vi "Process_Array.vi"(4 "Image array":dbl[][](array[numeric]), 6 "Base_name":string, 7 "Image In":T4, 8 "Bleed (mm)":dbl, 9 "Step (mm) 2":dbl, 10 "X dim + bleed (mm)":dbl, 11 "Y dim + bleed (mm)":dbl) -> (3 "Image array":dbl[][](array[numeric]), 5 "Image Out":T4)   [LabVIEW 2018]
uses:
  <vilib>/vision/Image Controls.llb/IMAQ Image.ctl
  <vilib>/vision/Pattern Matching.llb/IMAQ Curve Parameters.ctl
  <vilib>/vision/Shape Detection.llb/ShapeDetectionMatchOptions.ctl
  <vilib>/vision/Pattern Matching.llb/IMAQ Match Range Setting.ctl
  <vilib>/Utility/file.llb/Write Delimited Spreadsheet (DBL).vi
  <vilib>/vision/NI_Vision_Development_Module.lvlib
panel:
  in  "Match Options":T1 {"Range Settings"."Match Constraints" items=["Rotation Angle (degrees)", "Scale Factor (%)", "Occlusion (%)"]}
  in  "Curve Parameters":T3={"Extraction Mode"=0, "Edge Threshold"=75, "Edge Filter Size"=1, "Min Length"=25, "Row Search Step Size"=15, "Col Search Step Size"=15, "Max Endpoint Gap"=10, "Closed"=FALSE, "Subpixel"=FALSE} {"Max Endpoint Gap" min=0; "Col Search Step Size" min=1 max=255 step=1; "Row Search Step Size" min=1 max=255 step=1; "Min Length" min=0; "Edge Filter Size" items=["Fine", "Normal", "Controur Tracing"]; "Edge Threshold" min=1 max=65535 step=1; "Extraction Mode" items=["Normal", "Uniform Regions"]}
  out "Number of Matches Returned":i32
  # "Range"
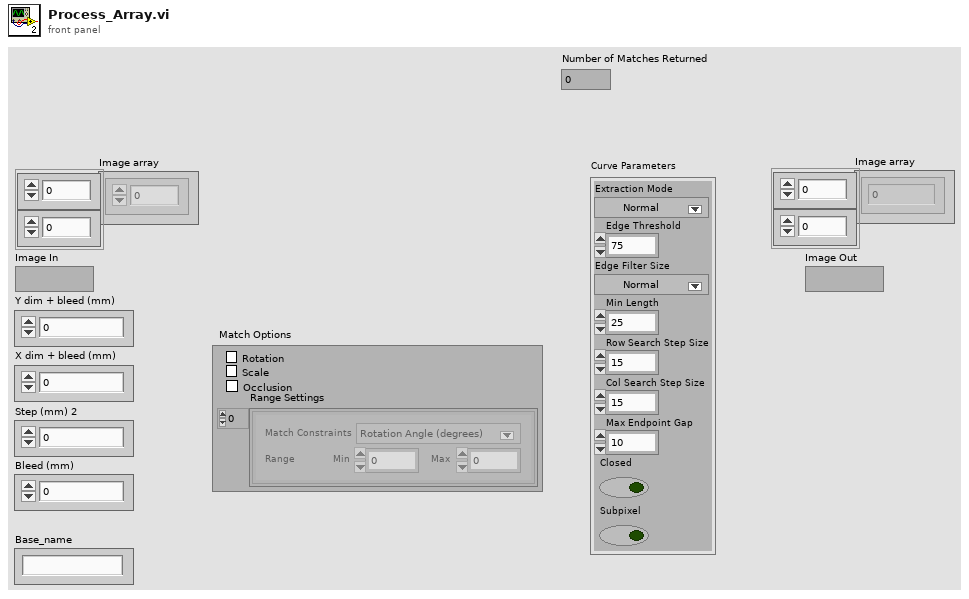
[diagram p1: front panel]
types:
  T1 = typedef "ShapeDetectionMatchOptions.ctl" = cluster{"Rotation":bool, "Scale":bool, "Occlusion":bool, "Range Settings":T2[]}
  T2 = typedef "IMAQ Match Range Setting.ctl" = cluster{"Match Constraints":u32, "Min":dbl, "Max":dbl}
  T3 = typedef "IMAQ Curve Parameters.ctl" = cluster{"Extraction Mode":u32, "Edge Threshold":i32, "Edge Filter Size":u32, "Min Length":i32, "Row Search Step Size":i32, "Col Search Step Size":i32, "Max Endpoint Gap":i32, "Closed":bool, "Subpixel":bool}
  T4 = typedef "IMAQ Image.ctl" = refnum<image>
  T5 = typedef "Image Type" = u32
  T6 = cluster{"Min Width":dbl, "Max Width":dbl, "Min Height":dbl, "Max Height":dbl}
  T7 = cluster{"Corners":cluster{"X":sgl, "Y":sgl}[], "Angle":dbl, "Width":dbl, "Height":dbl, "Score":dbl}[]
  T8 = typedef "ROI Descriptor" = cluster{"Global Rectangle":i32[], "Contours":cluster{"ID":enum32{"External", "Internal"}, "Type":u32, "Coordinates":i32[]}[]}
  T9 = cluster{"Corners":cluster{"X":sgl, "Y":sgl}[], "Angle":dbl, "Width":dbl, "Height":dbl, "Score":dbl}
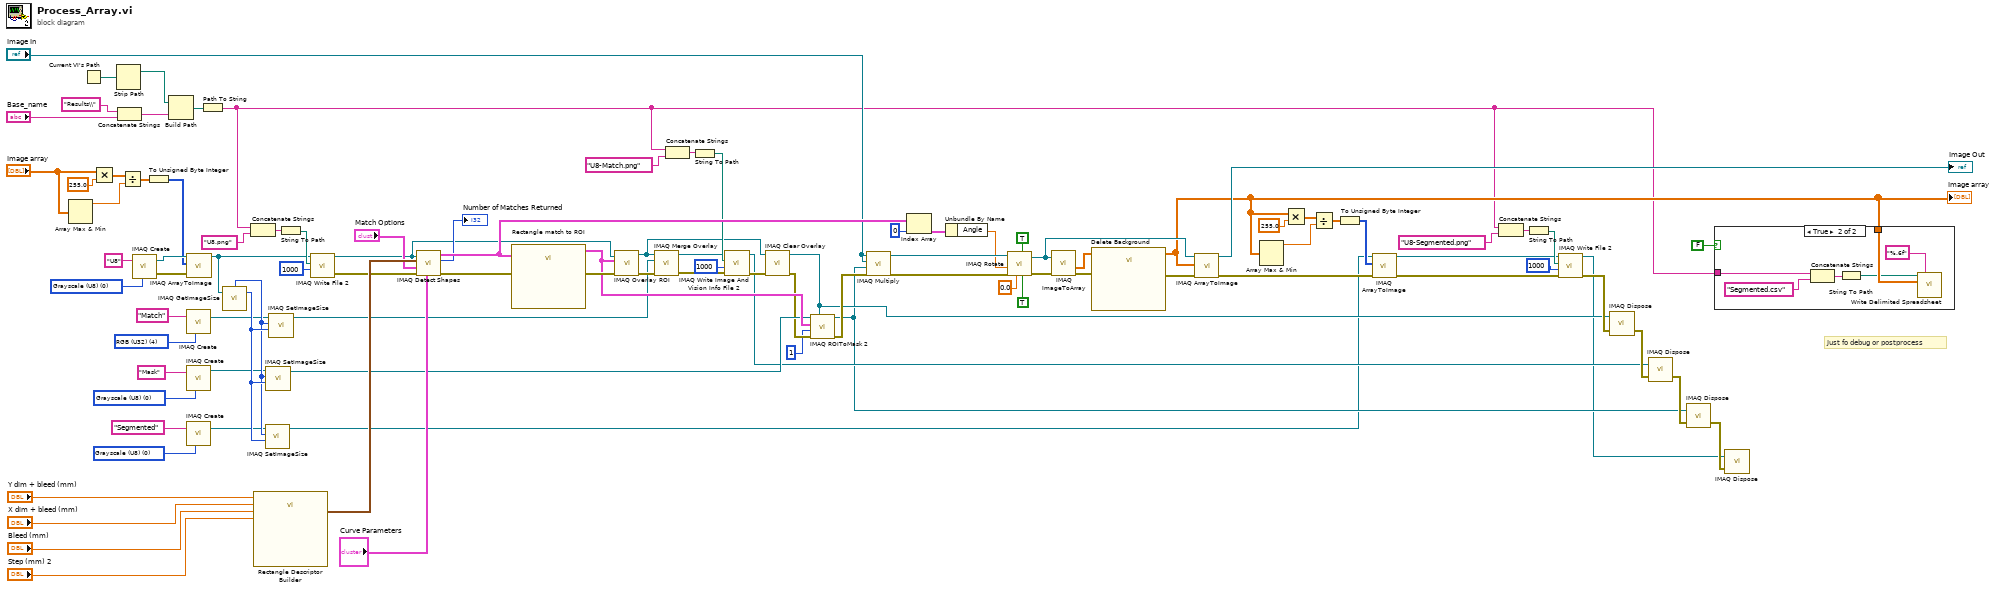
[diagram p0: block diagram]
diagram:
  w42 = T5 0 items=["Grayscale (U8)", "Grayscale (I16)", "Grayscale (SGL)", "Complex (CSG)", "RGB (U32)", "HSL (U32)", "RGB (U64)", "Grayscale (U16)"] ("Image Type")
  w44 = T5 4 items=["Grayscale (U8)", "Grayscale (I16)", "Grayscale (SGL)", "Complex (CSG)", "RGB (U32)", "HSL (U32)", "RGB (U64)", "Grayscale (U16)"] ("Image Type")
  w47 = T5 0 items=["Grayscale (U8)", "Grayscale (I16)", "Grayscale (SGL)", "Complex (CSG)", "RGB (U32)", "HSL (U32)", "RGB (U64)", "Grayscale (U16)"] ("Image Type")
  w98 = T5 0 items=["Grayscale (U8)", "Grayscale (I16)", "Grayscale (SGL)", "Complex (CSG)", "RGB (U32)", "HSL (U32)", "RGB (U64)", "Grayscale (U16)"] ("Image Type")
  # "Just fo debug or postprocess"
  n1 = Array Max & Min(array="Image array") -> (max value=w76:dbl)  [unwired: 3 out]
  n2 = Current VI's Path() -> (path=w58:path)
  n3 = Multiply(x="Image array", y=255.0) -> (x*y=w77:dbl[][])
  n4 = Strip Path(path=w58) -> (stripped path=w57:path)  [unwired: 1 out]
  n5 = Concatenate Strings("Results\\" ("name or relative path"), "Base_name") -> (w92:string)
  n6 = Divide(x=w77, y=w76) -> (x/y=w75:dbl[][])
  n7 = call "IMAQ Create"("Image Name"="U8", "Image Type"=w98) -> ("New Image"=w73:T4, "error out"=w74:errorcluster)  [unwired: 3 in]
  n8 = To Unsigned Byte Integer(number=w75) -> (unsigned 8bit integer=w72:u8[][])
  n9 = Build Path(base path=w57, name or relative path=w92) -> (appended path=w66:path)
  n10 = call "IMAQ Create"("Image Name"="Match", "Image Type"=w44) -> ("New Image"=w39:T4)  [unwired: 3 in, 1 out]
  n11 = call "IMAQ Create"("Image Name"="Mask", "Image Type"=w47) -> ("New Image"=w38:T4)  [unwired: 3 in, 1 out]
  n12 = call "IMAQ Create"("Image Name"="Segmented", "Image Type"=w42) -> ("New Image"=w37:T4)  [unwired: 3 in, 1 out]
  n13 = call "IMAQ ArrayToImage"("error in (no error)"=w74, "Image Pixels (U8)"=w72, "Image"=w73) -> ("Image Out"=w31:T4)  [unwired: 7 in, 1 out]
  n14 = Path To String(path=w66) -> (string=w2:string)
  n15 = call "IMAQ GetImageSize"("Image"=w31) -> ("Y Resolution"=w41:i32, "X Resolution"=w40:i32)  [unwired: 3 in, 1 out]
  n16 = Concatenate Strings(w2, "U8.png" ("string")) -> (w65:string)
  n17 = call "Rectangle Descriptor Builder.vi"("Step (mm) in"="Step (mm) 2", "Bleed (mm)"="Bleed (mm)", "X dim + bleed (mm)"="X dim + bleed (mm)", "Y dim + bleed (mm)"="Y dim + bleed (mm)") -> ("Rectangle Descriptor"=w70:T6)  [unwired: 7 in]
  n18 = call "IMAQ SetImageSize"("Y Resolution"=w41, "X Resolution"=w40, "Image"=w37) -> ("Image Out"=w5:T4)  [unwired: 2 in, 1 out]
  n19 = call "IMAQ SetImageSize"("Y Resolution"=w41, "X Resolution"=w40, "Image"=w38) -> ("Image Out"=w35:T4)  [unwired: 2 in, 1 out]
  n20 = call "IMAQ SetImageSize"("Y Resolution"=w41, "X Resolution"=w40, "Image"=w39) -> ("Image Out"=w36:T4)  [unwired: 2 in, 1 out]
  n21 = String To Path(string=w65) -> (path=w64:path)
  n22 = call-poly "IMAQ Write File 2"("Image Quality"=u32 1000, "File Path"=w64, "Image"=w31) -> ("error out"=w62:errorcluster, "Image Out (duplicate)"=w59:T4)  [unwired: 7 in]
  n23 = call-poly "IMAQ Detect Shapes"("Curve Parameters"="Curve Parameters", "error in (no error)"=w62, "Match Options"="Match Options", "Rectangle Descriptor"=w70, "Image"=w59) -> ("error out"=w95:errorcluster, "Number of Matches Returned"=→"Number of Matches Returned":i32, "Rectangles"=w87:T7)  [unwired: 4 in]
  n24 = call "Rectangle match to ROI.vi"("error in (no error)"=w95, "Rectangles"=w87) -> ("error out"=w94:errorcluster, "ROI Descriptor"=w46:T8)  [unwired: 8 in]
  n25 = call "IMAQ Overlay ROI"("error in (no error)"=w94, "ROI Descriptor"=w46, "Image"=w59) -> ("error out"=w53:errorcluster, "Image Out"=w50:T4)  [unwired: 7 in]
  n26 = call "IMAQ Merge Overlay"("error in (no error)"=w53, "Image Dst"=w36, "Image Src"=w50) -> ("error out"=w52:errorcluster, "Image Dst Out"=w51:T4)  [unwired: 7 in]
  n27 = Concatenate Strings(w2, "U8-Match.png" ("string")) -> (w61:string)
  n28 = String To Path(string=w61) -> (path=w56:path)
  n29 = call "IMAQ Write Image And Vision Info File 2"("error in (no error)"=w52, "Image Quality"=u32 1000, "File Path"=w56, "Image"=w51) -> ("error out"=w49:errorcluster, "Image Out (duplicate)"=w9:T4)  [unwired: 6 in]
  n30 = call "IMAQ Clear Overlay"("error in (no error)"=w49, "Image"=w50) -> ("error out"=w34:errorcluster, "Image Out"=w8:T4)  [unwired: 8 in]
  n31 = call "IMAQ ROIToMask 2"("Image Model"=w8, "error in (no error)"=w34, "Filling Value (255)"=1, "ROI Descriptor"=w46, "Image"=w35) -> ("error out"=w90:errorcluster, "Image Out"=w7:T4)  [unwired: 4 in, 1 out]
  n32 = call "IMAQ Multiply"("Image Src A"="Image In", "Image Dst"="Image In", "Image Src B"=w7, "error in (no error)"=w90) -> ("Image Dst Out"=w32:T4, "error out"=w89:errorcluster)  [unwired: 3 in]
  n33 = Index Array(array=w87, index=0) -> (element=w85:T9)
  n34 = Unbundle By Name(w85) -> ("Angle"=w30:dbl)
  n35 = call "IMAQ Rotate"("Use Bilinear Interpolation"=TRUE, "Maintain Size"=TRUE, "Replace Value"=sgl 0.0, "error in (no error)"=w89, "Angle (degrees)"=w30, "Image Src"=w32) -> ("error out"=w82:errorcluster, "Image Dst Out"=w29:T4)  [unwired: 4 in]
  n36 = call "IMAQ ImageToArray"("error in (no error)"=w82, "Image"=w29) -> ("Image Pixels (Float)"=w81:sgl[][], "error out"=w28:errorcluster)  [unwired: 2 in, 3 out]
  n37 = call "Delete Background.vi"("error in"=w28, "Image Pixels (Float) in"=w81) -> ("error out"=w27:errorcluster, "Image Pixels (Float) out"=w3:sgl[][])  [unwired: 8 in]
  "Image array" <- w3
  n38 = call "IMAQ ArrayToImage"("Image Pixels (Float)"=w3, "error in (no error)"=w27, "Image"=w29) -> ("error out"=w15:errorcluster, "Image Out"=→"Image Out":T4)  [unwired: 7 in]
  n39 = Array Max & Min(array=w3) -> (max value=w23:sgl)  [unwired: 3 out]
  n40 = Multiply(x=w3, y=255.0) -> (x*y=w24:dbl[][])
  n41 = Divide(x=w24, y=w23) -> (x/y=w22:dbl[][])
  n42 = To Unsigned Byte Integer(number=w22) -> (unsigned 8bit integer=w16:u8[][])
  n43 = call "IMAQ ArrayToImage"("error in (no error)"=w15, "Image Pixels (U8)"=w16, "Image"=w5) -> ("error out"=w14:errorcluster, "Image Out"=w17:T4)  [unwired: 7 in]
  n44 = Concatenate Strings(w2, "U8-Segmented.png" ("string")) -> (w21:string)
  n45 = String To Path(string=w21) -> (path=w20:path)
  n46 = call-poly "IMAQ Write File 2"("error in (no error)"=w14, "Image Quality"=u32 1000, "File Path"=w20, "Image"=w17) -> ("error out"=w13:errorcluster, "Image Out (duplicate)"=w6:T4)  [unwired: 6 in]
  n47 = call "IMAQ Dispose"("Image"=w8, "error in (no error)"=w13) -> ("error out"=w12:errorcluster)  [unwired: 4 in]
  n48 = call "IMAQ Dispose"("Image"=w9, "error in (no error)"=w12) -> ("error out"=w11:errorcluster)  [unwired: 4 in]
  n49 = call "IMAQ Dispose"("Image"=w7, "error in (no error)"=w11) -> ("error out"=w10:errorcluster)  [unwired: 4 in]
  n50 = case shown="True" FALSE {
    tunnel: w3 -> [_ w103]
    tunnel: w2 -> [_ w102]
    frame False {
    }
    frame True {
      n51 = Concatenate Strings(w102, "Segmented.csv" ("string")) -> (w101:string)
      n52 = String To Path(string=w101) -> (path=w100:path)
      n53 = call-poly <vilib>:"Write Delimited Spreadsheet.vi"("file path (dialog if empty)"=w100, "format (%.3f)"="%.6f", "2D data"=w103) -> ()  [unwired: 11 in, 2 out]
    }
  }
  n54 = call "IMAQ Dispose"("Image"=w6, "error in (no error)"=w10) -> ()  [unwired: 4 in, 1 out]
